vi "GdsLanguage_GetLanguagesStatus.vi"(5 "error in (no error)":errorcluster) -> (14 "SelectedLanguage":T1=enum."en", 15 "NoOfTranslatedStrings":i32, 16 "FoundLanguages":T1[](array[typedef]), 19 "error out":errorcluster)   [LabVIEW 2020]
doc: "Sets the current and backup languages, validates these languages (checks that \nthere are non-empty strings for all StringID entries), and load the translated strings into class memory for later use in the application."
uses:
  <resource>/Framework/Providers/Open_GDS/ClassProviders/Common/GdsLanguage/GdsLanguage_LanguageID.ctl
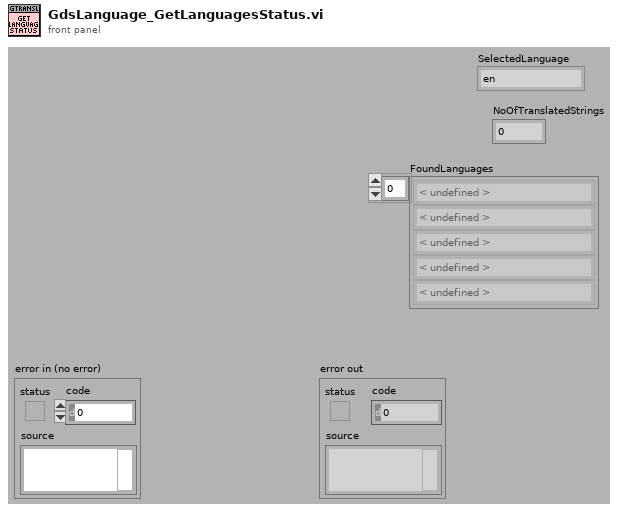
[diagram p1: front panel]
types:
  T1 = typedef "GdsLanguage_LanguageID.ctl" = enum16{"< undefined >", "aa", "ab", "af", "am", "ar", "as", "ay", "az", "ba", "be", "bg", "bh", "bi", "bn", "bo", "br", "ca", "co", "cs", "cy", "da", "de", "dz", "el", "en", "eo", "es", "et", "eu", "fa", "fi", "fj", "fo", "fr", "fy", "ga", "gd", "gl", "gn", "gu", "gv", "ha", "he", "hi", "hr", "hu", "hy", "ia", "id", "ie", "ik", "is", "it", "iu", "ja", "jv", "ka", "kk", "kl", "km", "kn", "ko", "ks", "ku", "ky", "la", "li", "ln", "lo", "lt", "lv", "mg", "mi", "mk", "ml", "mn", "mo", "mr", "ms", "mt", "my", "na", "ne", "nl", "no", "oc", "om", "or", "pa", "pl", "ps", "pt", "qu", "rm", "rn", "ro", "ru", "rw", "sa", "sd", "sg", "sh", "si", "sk", "sl", "sm", "sn", "so", "sq", "sr", "ss", "st", "su", "sv", "sw", "ta", "te", "tg", "th", "ti", "tk", "tl", "tn", "to", "tr", "ts", "tt", "tw", "ug", "uk", "ur", "uz", "vi", "vo", "wo", "xh", "yi", "yo", "zh", "zu"}
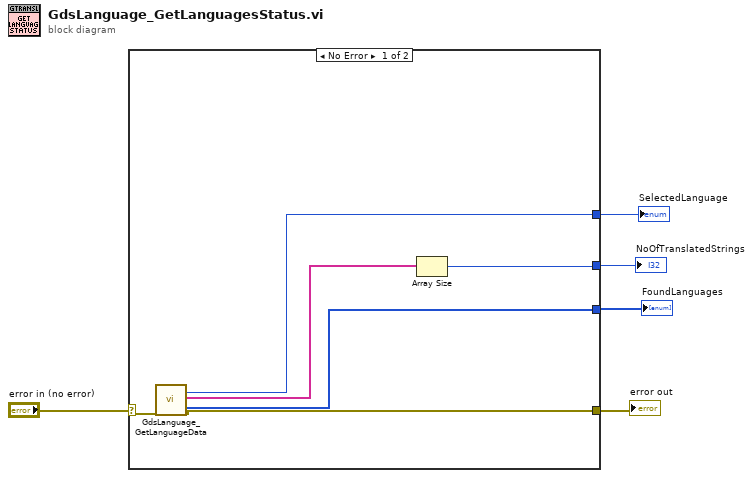
[diagram p0: block diagram]
diagram:
  n1 = case shown="No Error" "error in (no error)" {
    selector: "error in (no error)" -> [w10 w12]
    tunnel: [w9 w12] -> w4
    tunnel: [w8 _] -> w1
    tunnel: [w11 _] -> w3
    tunnel: [w6 _] -> w2
    frame No Error {
      n2 = call <resource>:"GdsLanguage_GetLanguageData.vi"("error in (no error)"=w10) -> ("Language"=w6:T1, "StringIDArray"=w7:string[], "FoundLanguages"=w8:T1[], "error out"=w9:errorcluster)  [unwired: 14 in, 1 out]
      n3 = Array Size(array=w7) -> (size(s)=w11:i32)
    }
    frame Error {
    }
  }
  "error out" <- w4
  "SelectedLanguage" <- w2
  "NoOfTranslatedStrings" <- w3
  "FoundLanguages" <- w1
